vi "Shutdown.vi"(8 "error in (no error)":errorcluster, 11 "Process in":refnum<class "Process.lvclass">) -> (0 "error out":errorcluster)   [LabVIEW 2019, in "TimingDRV Engine.lvlib" / "Process.lvclass"]
uses:
  Process.lvclass
  Process.lvclass/Process.ctl
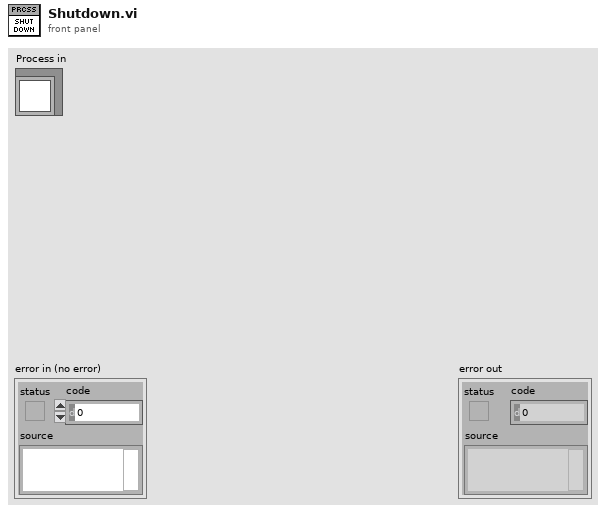
[diagram p1: front panel]
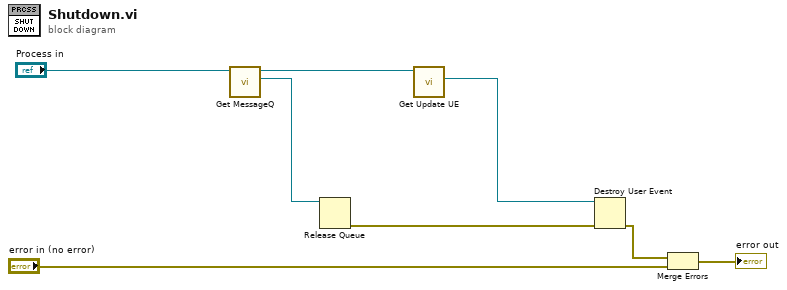
[diagram p0: block diagram]
diagram:
  n1 = call "Get MessageQ.vi"("CD_Process in"="Process in") -> ("MessageQ"=w7:refnum<queue>, "CD_Process out"=w6:refnum<class "Process.lvclass">)  [unwired: 9 in]
  n2 = Release Queue(queue=w7) -> (error out=w5:errorcluster)  [unwired: 2 in, 2 out]
  n3 = call "Get Update UE.vi"("CD_Process in"=w6) -> ("Update UE"=w4:refnum<user-event>)  [unwired: 9 in, 1 out]
  n4 = Destroy User Event(user event=w4, error in=w5) -> (error out=w3:errorcluster)
  n5 = Merge Errors(w3, "error in (no error)") -> (→"error out":errorcluster)
